vi "read dummy register accelerometer.vi"() -> ()   [LabVIEW 2019]
panel:
  out "data's booleans":bool[](array[boolean])
  out "read data":u8 format="%x"
  out "ACK3":bool
  out "SDA3":bool
  out "SDA2":bool
  out "ACK2":bool
  out "SDA1":bool
  out "ACK1":bool
  in  "add + read bite":u8 format="%x"
  in  "register":u8 format="%x"
  in  "adresse + Write":u8 format="%x"
  out "adress + READ booleans":bool[](array[boolean])
  out "register adress":bool[](array[boolean])
  out "Adresse + command byte":bool[](array[boolean])
  # "hex"
  # "decimal"
  # "51"
  # "33"
  # "32"
  # "50"
  # "0F"
  # "15"
  # "expected data :"
  # "00110011"
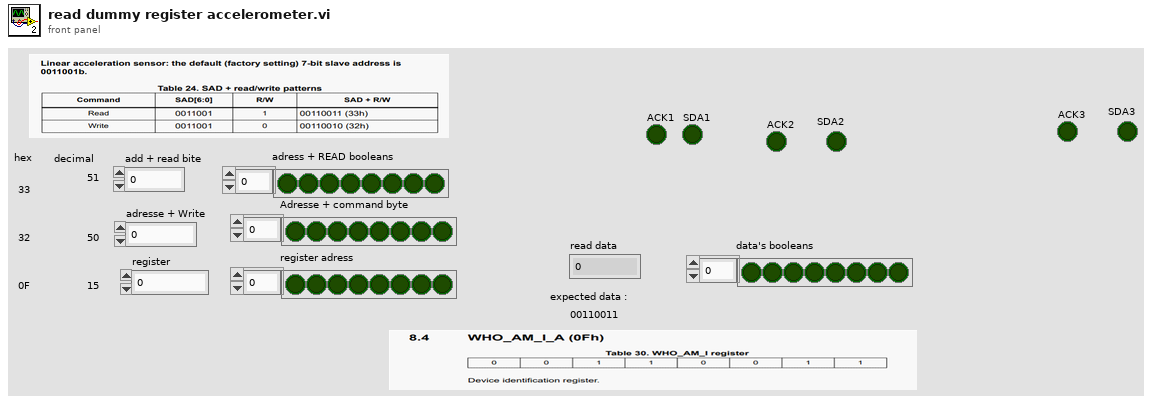
[diagram p1: front panel]
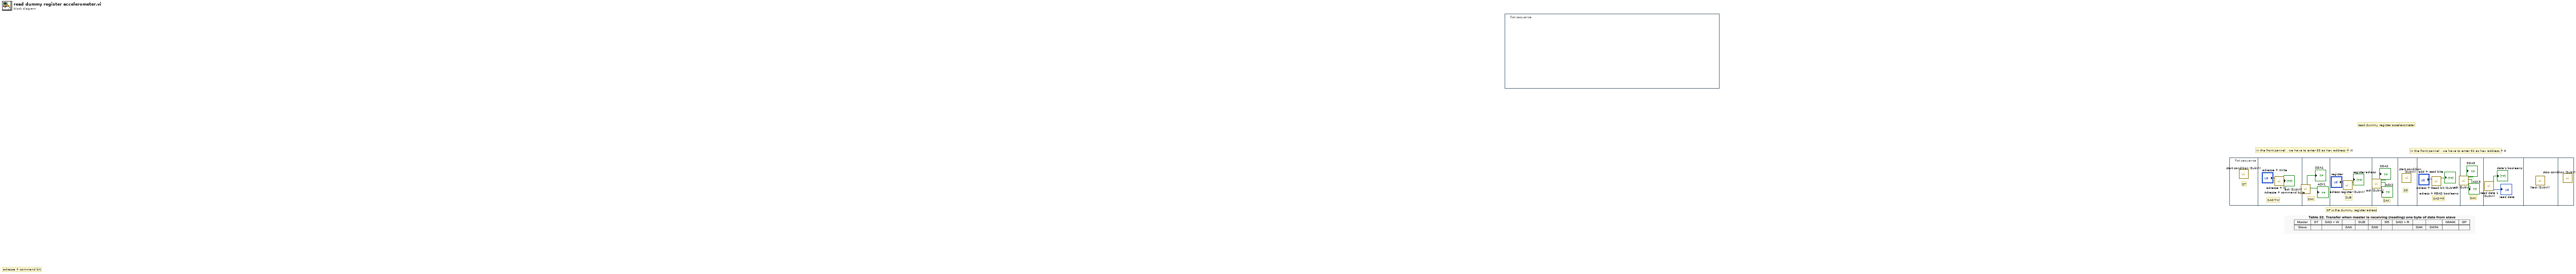
[diagram p0: block diagram]
diagram:
  # "0F is the dummy register adress"
  # "in the front pannel , we have to enter 32 as hex address + R"
  # "read dummy register accelerometer"
  # "in the front pannel , we have to enter 33 as hex address + W"
  # "adresse + command bit"
  n1 = flat-sequence {
    frame #0 {
    }
  }
  n2 = flat-sequence {
    frame #0 {
      # "ST"
      n3 = call "start condition (SubVI).vi"() -> ()  [unwired: 12 in]
    }
    frame #1 {
      # "SAD+W"
      n4 = call "adresse + W.vi"("adresse + Write"="adresse + Write") -> ("Adresse + command byte"=→"Adresse + command byte":bool[])  [unwired: 10 in]
    }
    frame #2 {
      # "SAK"
      n5 = call "ack (SubVI).vi"() -> ("ACK"=→"ACK1":bool, "SDA"=→"SDA1":bool)  [unwired: 10 in]
    }
    frame #3 {
      # "SUB"
      n6 = call "adress register (SubVI).vi"("register"="register") -> ("register adress"=→"register adress":bool[])  [unwired: 10 in]
    }
    frame #4 {
      # "SAK"
      n7 = call "ack (SubVI).vi"() -> ("ACK"=→"ACK2":bool, "SDA"=→"SDA2":bool)  [unwired: 10 in]
    }
    frame #5 {
      # "SR"
      n8 = call "start condition (SubVI).vi"() -> ()  [unwired: 12 in]
    }
    frame #6 {
      # "SAD+R"
      n9 = call "adress + Read bit (SubVI).vi"("add + read bite"="add + read bite") -> ("adress + R booleans"=→"adress + READ booleans":bool[])  [unwired: 10 in]
    }
    frame #7 {
      # "SAK"
      n10 = call "ack (SubVI).vi"() -> ("ACK"=→"ACK3":bool, "SDA"=→"SDA3":bool)  [unwired: 10 in]
    }
    frame #8 {
      n11 = call "read data 1  (SubVI).vi"() -> ("read data"=→"read data":u8, "data's booleans"=→"data's booleans":bool[])  [unwired: 10 in]
    }
    frame #9 {
      n12 = call "Nack (SubVI).vi"() -> ()  [unwired: 12 in]
    }
    frame #10 {
      n13 = call "stop condtion (SubVI).vi"() -> ()  [unwired: 12 in]
    }
  }
